vi "ge_MeasEnum2String.vi"(5 "MeasType":T1=enum."Dynamic") -> (2 "MeasType":string)   [LabVIEW 2011]
uses:
  Custom Ctrls/ge_MeasType.ctl
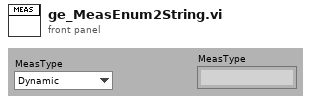
[diagram p1: front panel]
types:
  T1 = typedef "ge_MeasType.ctl" = enum16{"Voltage", "Frequency", "Tachometer", "Dynamic", "Thermocouple", "RTD", "Strain", "Current", "Resistance"}
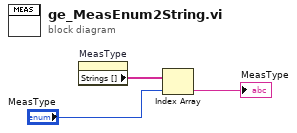
[diagram p0: block diagram]
diagram:
  n1 = property on="MeasType" class="Enum (strict)"() -> ("Strings []"=w3:string[])  [unwired: 2 in, 2 out]
  n2 = Index Array(array=w3, index="MeasType") -> (element=→"MeasType":string)
